vi "Write File Path.vi"(8 "error in (no error)":errorcluster, 10 "File Path":path, 11 "File Path Result in":refnum<class "File Path Result.lvclass">) -> (0 "error out":errorcluster, 3 "File Path Result out":refnum<class "File Path Result.lvclass">)   [LabVIEW 2015, in "File Path Result.lvclass"]
uses:
  File Path Result.lvclass
  File Path Result.lvclass/File Path Result.ctl
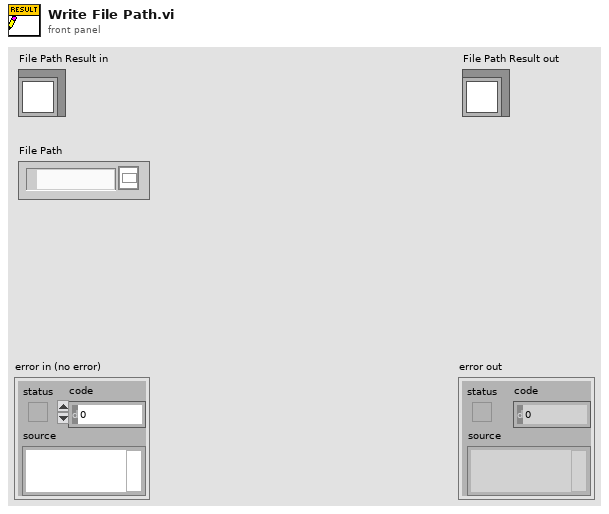
[diagram p1: front panel]
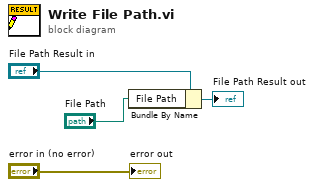
[diagram p0: block diagram]
diagram:
  n1 = Bundle By Name(cluster="File Path Result in", "File Path"="File Path") -> (→"File Path Result out":refnum<class "File Path Result.lvclass">)
  "error out" <- "error in (no error)"
